vi "Destroy.vi"(11 "AF Queue Stream in":refnum<class "AF Queue Stream.lvclass">) -> ()   [LabVIEW 2020, in "AF Queue Stream.lvclass"]
uses:
  AF Queue Stream.lvclass
  <vilib>/ActorFramework/Message Queue/Message Queue.lvclass
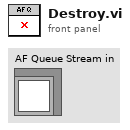
[diagram p1: front panel]
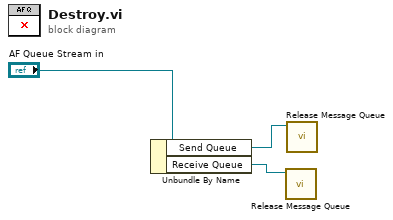
[diagram p0: block diagram]
diagram:
  n1 = Unbundle By Name("AF Queue Stream in") -> ("Send Queue"=w1:refnum<class "Message Queue.lvclass">, "Receive Queue"=w2:refnum<class "Message Queue.lvclass">)
  n2 = call <vilib>:"Release Message Queue.vi"("Message Queue"=w2) -> ()  [unwired: 9 in, 2 out]
  n3 = call <vilib>:"Release Message Queue.vi"("Message Queue"=w1) -> ()  [unwired: 9 in, 2 out]
